vi "Setup FP Data.vi"(8 "Error":errorcluster, 9 "WkSpace":T1, 11 "FP":refnum<class "FP.lvclass">) -> (0 "Error Out":errorcluster, 3 "FP Out":refnum<class "FP.lvclass">)   [LabVIEW 2024, in "FP.lvclass"]
uses:
  FP.lvclass
  <vilib>/Utility/miscctls.llb/LVRectTypeDef.ctl
  FP.lvclass/FP.ctl
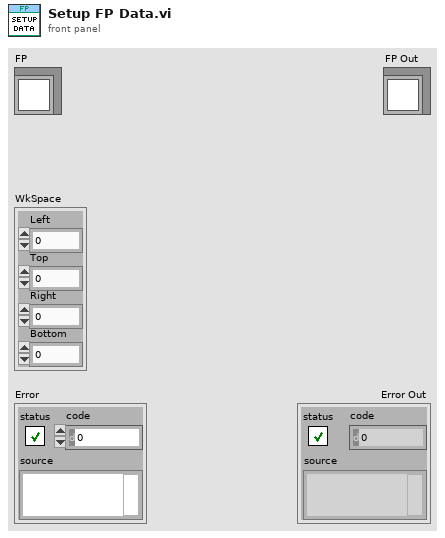
[diagram p1: front panel]
types:
  T1 = typedef "LVRectTypeDef.ctl" = cluster{"Left":i16, "Top":i16, "Right":i16, "Bottom":i16}
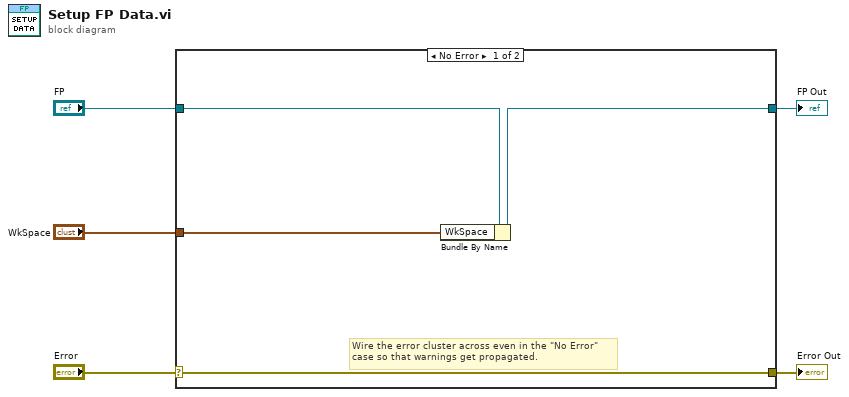
[diagram p0: block diagram]
diagram:
  n1 = case shown="No Error" "Error" {
    selector: "Error" -> [w9 w11]
    tunnel: [w9 w11] -> w4
    tunnel: [w7 w10] -> w2
    tunnel: "FP" -> [w8 w10]
    tunnel: "WkSpace" -> [w6 _]
    frame No Error {
      # "Wire the error cluster across even in the \"No Error\"\ncase so that warnings get propagated."
      n2 = Bundle By Name(cluster=w8, "WkSpace"=w6) -> (w7:refnum<class "FP.lvclass">)
    }
    frame Error {
    }
  }
  "Error Out" <- w4
  "FP Out" <- w2
